vi "SetupScope.vi"(4 "Record Length":i32=10000 format="%.0p", 6 "Sample Rate":dbl=5000000.0 format="%#.2p", 8 "error in (no error)":errorcluster, 10 "Reference Position":dbl=50.0 caption="Ref Position" format="%#.1f", 11 "IVI Refnum in":refnum<k15>) -> (0 "error out":errorcluster, 2 "channel name":string, 3 "IVI Refnum out":refnum<k15>)   [LabVIEW 2023]
uses:
  <instrlib>/niScope/Utility/niScope Get Channel Name From String.vi
  <instrlib>/niScope/Controls/niScope clock sync pulse source.ctl
  <resource>/objmgr/sessionReference.rc
  <instrlib>/niScope/Controls/niScope array measurement.ctl
  <instrlib>/niScope/Acquire/Fetch/niScope Fetch Complex WDT.vi
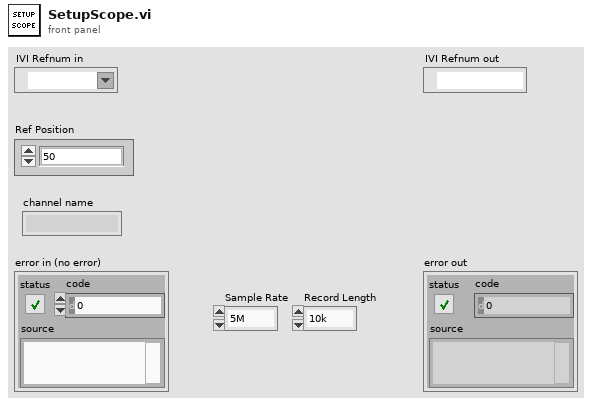
[diagram p1: front panel]
types:
  T1 = typedef "niScope array measurement.ctl" = i32
  T2 = typedef "niScope clock sync pulse source.ctl" = u16
  T3 = cluster{"actualSamples":i32, "absoluteInitialX":dbl, "relativeInitialX":dbl, "xIncrement":dbl, "offset":dbl, "gain":dbl, "reserved1":dbl, "reserved2":dbl}
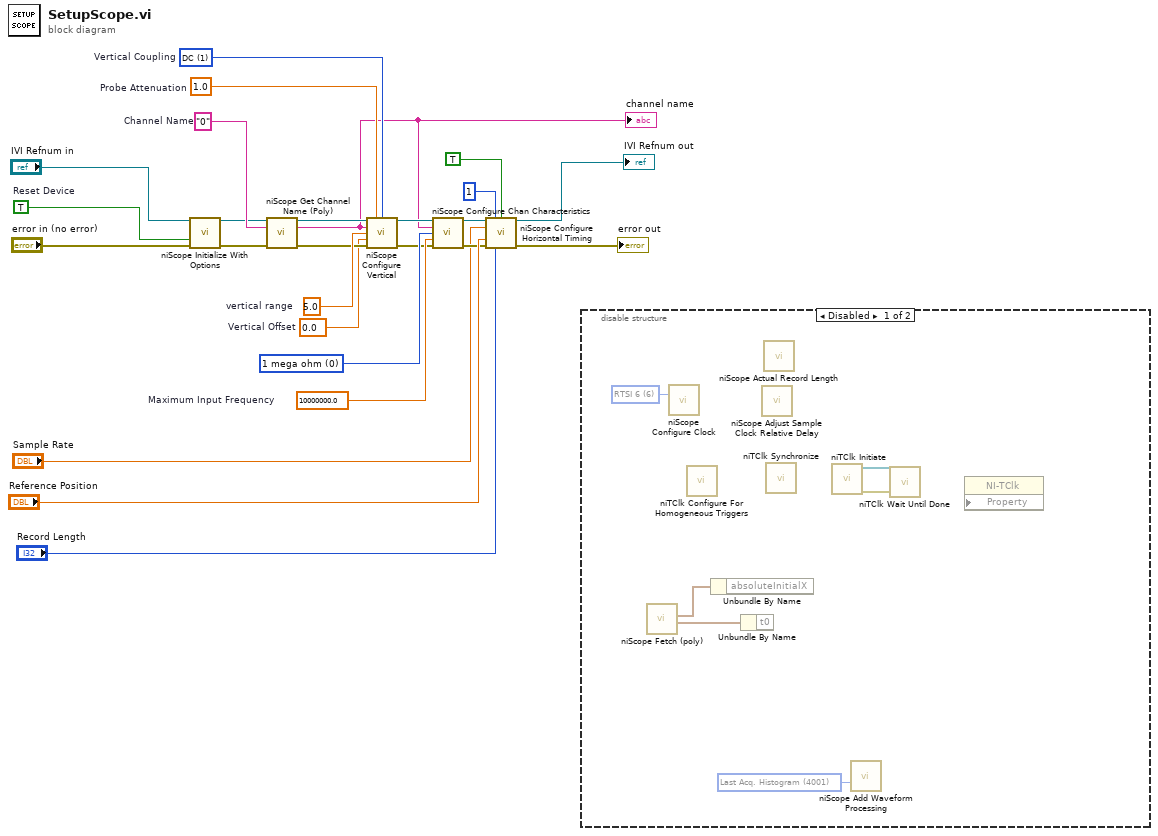
[diagram p0: block diagram]
diagram:
  w26 = "0"  # Channel Name
  w15 = 1.0  # Probe Attenuation
  w16 = 10000000.0  # Maximum Input Frequency
  w17 = 1 items=["AC", "DC", "Ground"]  # Vertical Coupling
  w14 = 0.0  # Vertical Offset
  w22 = 5.0  # vertical range
  w21 = u32 0 items=["1 mega ohm"=0, "50 ohms"=2] ("input impedance")
  w5 = TRUE  # Reset Device
  n1 = call <instrlib>:"niScope Initialize With Options.vi"("resource name"="IVI Refnum in", "reset device"=w5, "error in"="error in (no error)") -> ("instrument handle"=w6:refnum<k15>, "error out"=w7:errorcluster)  [unwired: 11 in]
  n2 = call-poly <instrlib>:"niScope Get Channel Name (Poly).vi"("instrument handle"=w6, "index"=w26, "error in"=w7) -> ("instrument handle out"=w19:refnum<k15>, "channel name"=w2:string, "error out"=w20:errorcluster)  [unwired: 10 in]
  "channel name" <- w2
  n3 = call <instrlib>:"niScope Configure Vertical.vi"("instrument handle"=w19, "probe attenuation"=w15, "vertical coupling"=w17, "channels"=w2, "vertical range"=w22, "vertical offset"=w14, "error in"=w20) -> ("instrument handle out"=w10:refnum<k15>, "error out"=w11:errorcluster)  [unwired: 7 in]
  n4 = call <instrlib>:"niScope Configure Chan Characteristics.vi"("instrument handle"=w10, "channels"=w2, "input impedance"=w21, "maximum input frequency"=w16, "error in"=w11) -> ("instrument handle out"=w13:refnum<k15>, "error out"=w12:errorcluster)  [unwired: 9 in]
  n5 = call <instrlib>:"niScope Configure Horizontal Timing.vi"("instrument handle"=w13, "number of records"=1, "enforce realtime"=TRUE ("Enforce Realtime"), "min sample rate"="Sample Rate", "reference position"="Reference Position", "error in"=w12, "min record length"="Record Length") -> ("instrument handle out"=→"IVI Refnum out":refnum<k15>, "error out"=→"error out":errorcluster)  [unwired: 7 in]
  n6 = disable-structure shown="Disabled" {
    frame Disabled {
      w29 = T1 4001 items=["None"=4000, "Last Acq. Histogram"=4001, "Multi Acq. Voltage Histogram"=4004, "Multi Acq. Time Histogram"=4005, "Multi Acq. Average"=4016, "Polynomial Interpolation"=4011, "Array Integral"=4006, "Derivative"=4007, "Inverse"=4008, "Multiply Channels"=4012, "Add Channels"=4013, "Subtract Channels"=4014, "Divide Channels"=4015, "Array Offset"=4025, "Array Gain"=4026, "Hanning Window"=4009, "Flat Top Window"=4010, "Hamming Window"=4020, "Triangle Window"=4023, "Blackman Window"=4024, "FIR Windowed Filter"=4021, "Bessel IIR Filter"=4022, "Butterworth IIR Filter"=4017, "Chebyshev IIR Filter"=4018, "FFT Phase Spectrum"=4002, "FFT Amp. Spectrum (Volts RMS)"=4003, "FFT Amp. Spectrum (dB)"=4019] ("array measurement")
      w32 = T2 6 items=["RTSI 0", "RTSI 1", "RTSI 2", "RTSI 3", "RTSI 4", "RTSI 5", "RTSI 6", "PFI 1", "PFI 2", "Internal"] ("clock sync pulse source")
      n7 = call-poly <instrlib>:"niScope Fetch (poly).vi"() -> ("wfm"=w27:waveform(cdb), "wfm info"=w28:T3)  [unwired: 8 in, 2 out]
      n8 = call <instrlib>:"niScope Configure Clock.vi"("clock sync pulse source"=w32) -> ()  [unwired: 13 in, 2 out]
      n9 = call <instrlib>:"niTClk Configure For Homogeneous Triggers.vi"() -> ()  [unwired: 10 in, 2 out]
      n10 = Unbundle By Name(w28) -> ()  [unwired: 1 out]
      n11 = Unbundle By Name(w27) -> ()  [unwired: 1 out]
      n12 = call <instrlib>:"niScope Adjust Sample Clock Relative Delay.vi"() -> ()  [unwired: 14 in, 2 out]
      n13 = call <instrlib>:"niScope Actual Record Length.vi"() -> ()  [unwired: 13 in, 3 out]
      n14 = call <instrlib>:"niTClk Synchronize.vi"() -> ()  [unwired: 10 in, 2 out]
      n15 = call <instrlib>:"niTClk Initiate.vi"() -> ("error out"=w31:errorcluster, "sessions out"=w30:refnum<k20>[])  [unwired: 10 in]
      n16 = call <instrlib>:"niScope Add Waveform Processing.vi"("array measurement"=w29) -> ()  [unwired: 13 in, 2 out]
      n17 = call <instrlib>:"niTClk Wait Until Done.vi"("error in (no error)"=w31, "sessions"=w30) -> ()  [unwired: 8 in, 2 out]
      n18 = property class="NI-TClk" props=[]() -> ()  [unwired: 3 in, 2 out]
    }
    frame Enabled {
    }
  }
